vi "SuperAuton-SlowCanGrab.vi"(8 "error in (no error)":errorcluster, 9 "TimeToPull":dbl, 11 "Auton Event Queue Data":refnum<queue>) -> (0 "error out":errorcluster, 2 "Success?":bool, 3 "Auton Event Queue Data 2":refnum<queue>)   [LabVIEW 2014]
uses:
  Robot Global Data.vi
  <vilib>/Rock Robotics/WPI/RobotDrive/WPI_RobotDriveGetSetRefNum.vi
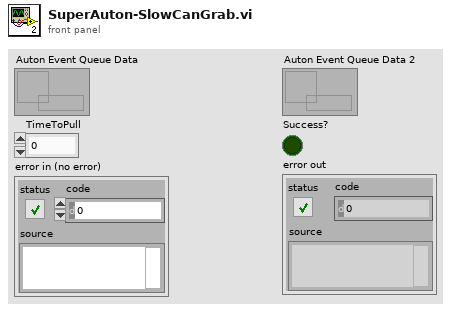
[diagram p1: front panel]
types:
  T1 = typedef "WPI_RobotDriveDevRef.ctl" = cluster{"DevStatus":errorcluster, "Motors[]":T2[], "Square Inputs":bool, "Max Output":dbl}
  T2 = typedef "WPI_MotorControlDeviceRef.ctl" = cluster{"DeviceStatus":errorcluster, "Type":T3, "PWM":cluster{"Controller":T4, "PWM Channel":T5, "DeadBand":T6}, "CAN":cluster{"Device Number":u8, "Control Mode":T7, "Semaphore":T8, "Max Vout":dbl, "TalonSRX Control Mode":T9}, "Invert":bool, "TransformRef":T10, "InvTransformRef":T10}
  T3 = typedef "WPI_MotorControlType.ctl" = enum16{"PWM", "CAN", "CANTalonSRX"}
  T4 = typedef "FPGA_TypedefDigitalModule.ctl" = enum16{"Controller 1"}
  T5 = typedef "FPGA_DIOPWMChannel.ctl" = enum8{"PWM 0", "PWM 1", "PWM 2", "PWM 3", "PWM 4", "PWM 5", "PWM 6", "PWM 7", "PWM 8", "PWM 9", "PWM MXP 0", "PWM MXP 1", "PWM MXP 2", "PWM MXP 3", "PWM MXP 4", "PWM MXP 5", "PWM MXP 6", "PWM MXP 7", "PWM MXP 8", "PWM MXP 9", "Invalid"}
  T6 = typedef "WPI_PWMDeadband.ctl" = cluster{"Name":string, "maxPositivePwm":i32, "minPositivePwm":i32, "centerPwm":i32, "maxNegativePwm":i32, "minNegativePwm":i32, "angularRange":u16}
  T7 = typedef "WPI_CANJaguar_ControlMode.ctl" = enum8{"Percent VBus", "Current", "Speed", "Position", "Voltage"}
  T8 = typedef "Semaphore RefNum" = refnum<k1>
  T9 = typedef "WPI_CANTalonSRX_APIControlMode.ctl" = enum8{"Percent VBus", "Speed", "Position", "Slave", "Unchanged / Invalid"}
  T10 = typedef "WPI_PWMTransform_ConPane.ctl" = refnum<vi>
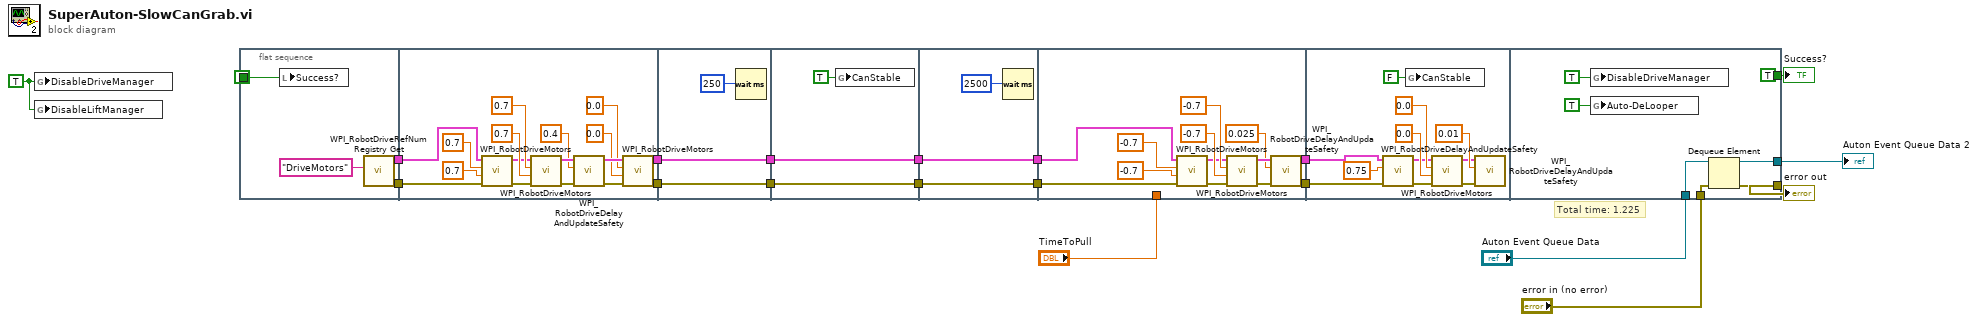
[diagram p0: block diagram]
diagram:
  w16 = TRUE ("Success?")
  # "Total time: 1.225"
  n1 = global write "Robot Global Data.vi" "DisableDriveManager"(w16) -> ()
  n2 = global write "Robot Global Data.vi" "DisableLiftManager"(w16) -> ()
  n3 = flat-sequence {
    tunnel: FALSE ("Success?") -> [w24]
    tunnel: [w22] -> w14
    tunnel: [w21] -> w15
    tunnel: w15 -> [w27]
    tunnel: w14 -> [w28]
    tunnel: [w41] -> w13
    tunnel: [w40] -> w12
    tunnel: w13 -> [w44]
    tunnel: [w44] -> w11
    tunnel: w12 -> [w43]
    tunnel: [w43] -> w10
    tunnel: w11 -> [w46]
    tunnel: w10 -> [w45]
    tunnel: [w46] -> w9
    tunnel: [w45] -> w8
    tunnel: [w49] -> w7
    tunnel: w9 -> [w49]
    tunnel: [w48] -> w6
    tunnel: w8 -> [w48]
    tunnel: "TimeToPull" -> [_]
    tunnel: w7 -> [w54]
    tunnel: w6 -> [w52]
    tunnel: [w58] -> w5
    tunnel: [w57] -> w4
    tunnel: w5 -> [w68]
    tunnel: w4 -> [w65]
    tunnel: [TRUE ("Success?")] -> w3
    tunnel: "Auton Event Queue Data" -> [w78]
    tunnel: "error in (no error)" -> [w77]
    tunnel: [w76] -> w18
    tunnel: [w75] -> w17
    frame #0 {
      n4 = local write "Success?"(w24) -> ()
      n5 = call <vilib>:"WPI_RobotDriveRefNum Registry Get.vi"("refnum name"="DriveMotors") -> ("error out"=w21:errorcluster, "RobotDriveDevRef"=w22:T1)  [unwired: 9 in]
    }
    frame #1 {
      n6 = call <vilib>:"WPI_RobotDriveMotors.vi"("error in (no error)"=w27, "RightSpeed"=0.7 ("Y axis value"), "LeftSpeed"=0.7 ("X axis value"), "RobotDriveDevRef"=w28) -> ("error out"=w25:errorcluster, "RobotDriveDevRef"=w26:T1)  [unwired: 5 in, 1 out]
      n7 = call <vilib>:"WPI_RobotDriveMotors.vi"("error in (no error)"=w25, "RightSpeed"=0.7 ("Y axis value"), "LeftSpeed"=0.7 ("X axis value"), "RobotDriveDevRef"=w26) -> ("error out"=w36:errorcluster, "RobotDriveDevRef"=w37:T1)  [unwired: 5 in, 1 out]
      n8 = call <vilib>:"WPI_RobotDriveDelayAndUpdateSafety.vi"("error in (no error)"=w36, "Delay (s)"=0.4, "RobotDriveDevRef"=w37) -> ("error out"=w33:errorcluster, "RobotDriveDevRef 2"=w34:T1)  [unwired: 7 in]
      n9 = call <vilib>:"WPI_RobotDriveMotors.vi"("error in (no error)"=w33, "RightSpeed"=0.0 ("Y axis value"), "LeftSpeed"=0.0 ("X axis value"), "RobotDriveDevRef"=w34) -> ("error out"=w40:errorcluster, "RobotDriveDevRef"=w41:T1)  [unwired: 5 in, 1 out]
    }
    frame #2 {
      n10 = Wait (ms)(milliseconds to wait=u32 250) -> ()  [unwired: 1 out]
    }
    frame #3 {
      n11 = global write "Robot Global Data.vi" "CanStable"(TRUE) -> ()
    }
    frame #4 {
      n12 = Wait (ms)(milliseconds to wait=u32 2500) -> ()  [unwired: 1 out]
    }
    frame #5 {
      n13 = call <vilib>:"WPI_RobotDriveMotors.vi"("error in (no error)"=w52, "RightSpeed"=-0.7 ("Y axis value"), "LeftSpeed"=-0.7 ("X axis value"), "RobotDriveDevRef"=w54) -> ("error out"=w51:errorcluster, "RobotDriveDevRef"=w53:T1)  [unwired: 5 in, 1 out]
      n14 = call <vilib>:"WPI_RobotDriveMotors.vi"("error in (no error)"=w51, "RightSpeed"=-0.7 ("Y axis value"), "LeftSpeed"=-0.7 ("X axis value"), "RobotDriveDevRef"=w53) -> ("error out"=w60:errorcluster, "RobotDriveDevRef"=w61:T1)  [unwired: 5 in, 1 out]
      n15 = call <vilib>:"WPI_RobotDriveDelayAndUpdateSafety.vi"("error in (no error)"=w60, "Delay (s)"=0.025, "RobotDriveDevRef"=w61) -> ("error out"=w57:errorcluster, "RobotDriveDevRef 2"=w58:T1)  [unwired: 7 in]
    }
    frame #6 {
      n16 = call <vilib>:"WPI_RobotDriveDelayAndUpdateSafety.vi"("error in (no error)"=w65, "Delay (s)"=0.75, "RobotDriveDevRef"=w68) -> ("error out"=w66:errorcluster, "RobotDriveDevRef 2"=w67:T1)  [unwired: 7 in]
      n17 = global write "Robot Global Data.vi" "CanStable"(FALSE) -> ()
      n18 = call <vilib>:"WPI_RobotDriveMotors.vi"("error in (no error)"=w66, "RightSpeed"=0.0 ("Y axis value"), "LeftSpeed"=0.0 ("X axis value"), "RobotDriveDevRef"=w67) -> ("error out"=w72:errorcluster, "RobotDriveDevRef"=w73:T1)  [unwired: 5 in, 1 out]
      n19 = call <vilib>:"WPI_RobotDriveDelayAndUpdateSafety.vi"("error in (no error)"=w72, "Delay (s)"=0.01, "RobotDriveDevRef"=w73) -> ()  [unwired: 7 in, 2 out]
    }
    frame #7 {
      n20 = global write "Robot Global Data.vi" "DisableDriveManager"(TRUE ("DisableDriveManager")) -> ()
      n21 = global write "Robot Global Data.vi" "Auto-DeLooper"(TRUE ("DisableDriveManager")) -> ()
      n22 = Dequeue Element(queue=w78, error in (no error)=w77) -> (queue out=w76:refnum<queue>, error out=w75:errorcluster)  [unwired: 1 in, 2 out]
    }
  }
  "error out" <- w17
  "Auton Event Queue Data 2" <- w18
  "Success?" <- w3
